vi "DQMH Build Module Disk Path From DQMH Path.vi"(8 "error in (no error)":errorcluster, 11 "Module DQMH Path":path) -> (0 "error out":errorcluster, 1 "Module Name":string, 2 "Clone ID":i32, 3 "Module Disk Path":path)   [LabVIEW 2022 SP3, in "hse-dqmh.lvlib"]
doc: "Parses the Instance Name for the Clone ID and returns the full path to the module's directory, the Clone ID and the module's name\n\n____\nHAMPEL SOFTWARE ENGINEERING v3.8.0 (2023-12-18 14:41)"
uses:
  hse-dqmh.lvlib
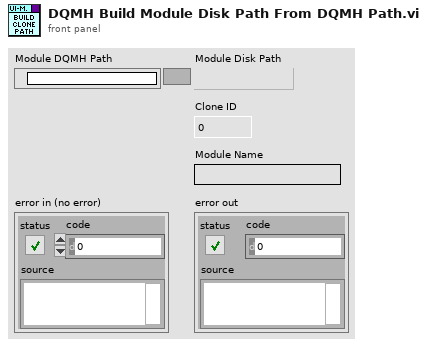
[diagram p1: front panel]
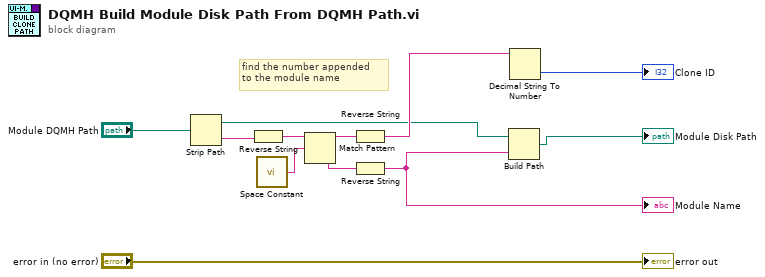
[diagram p0: block diagram]
diagram:
  # "find the number appended \nto the module name"
  n1 = Strip Path(path="Module DQMH Path") -> (stripped path=w2:path, name=w3:string)
  n2 = Reverse String(1:w3) -> (0:w10:string)
  n3 = call <vilib>:"Space Constant.vi"() -> ("String"=w9:string)
  n4 = Match Pattern(string=w10, regular expression=w9) -> (before substring=w6:string, after substring=w8:string)  [unwired: 1 in, 2 out]
  n5 = Reverse String(1:w6) -> (0:w4:string)
  n6 = Reverse String(1:w8) -> (0:w7:string)
  "Module Name" <- w7
  n7 = Build Path(base path=w2, name or relative path=w7) -> (appended path=→"Module Disk Path":path)
  n8 = Decimal String To Number(string=w4) -> (number=→"Clone ID":i32)  [unwired: 2 in, 1 out]
  "error out" <- "error in (no error)"
